vi "paste.vi"(2 "copyAry":string[][](array[string]), 3 "future event?":bool, 4 "Value":i32[](array[numeric]), 5 "ItemNames in":string[][](array[string])) -> (0 "val(sgnl)":i32[](array[numeric]), 1 "ItemNames out":string[][](array[string]))   [LabVIEW 2021]
panel:
  # "About This VI (pastes copied array to the LIST under highlighted cursor)\n- Pastes (inserts) copied array, called \"coppery\" underneath highlighted row of array \"ItemName in\" and outputs resulting array \"ItemNames out\"  \n\n*If highlighted cursor is located at the past event, it will send \"You cannot edit the current or past sequence.\" message.\n*Also, if highlighted cursor has multiple value, that is to say if multiple  lines are highlighted, it will send \"Select only one line  to add more.\" message."
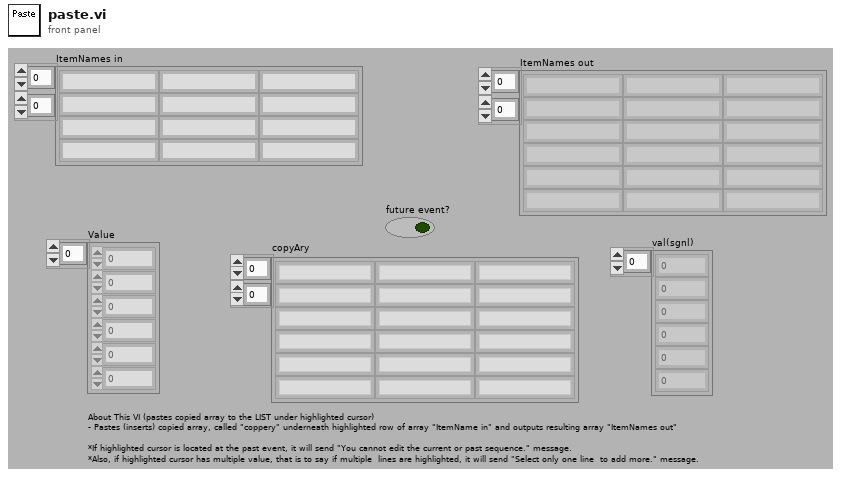
[diagram p1: front panel]
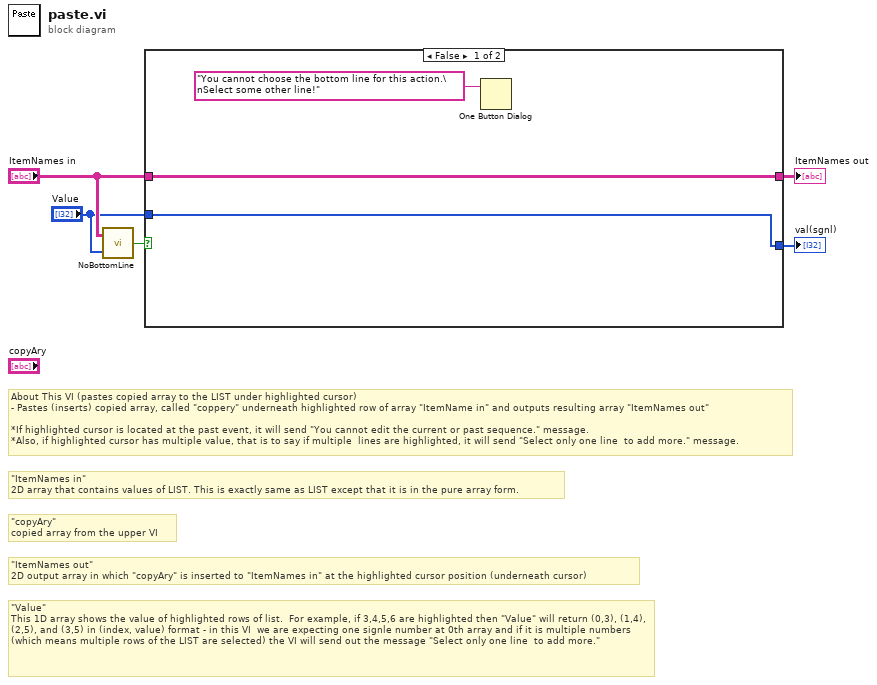
[diagram p0: block diagram]
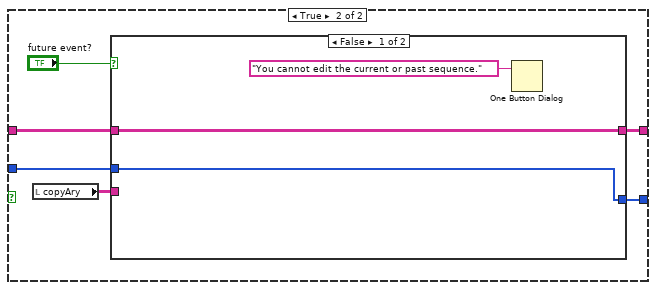
[diagram p2: hidden frame]
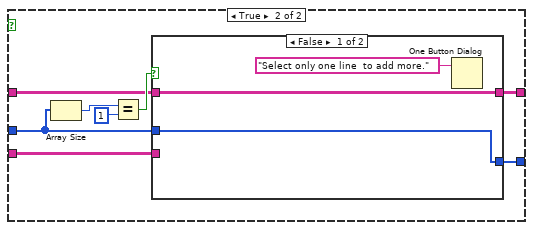
[diagram p3: hidden frame]
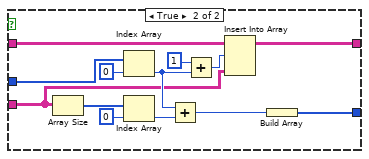
[diagram p4: hidden frame]
diagram:
  # "About This VI (pastes copied array to the LIST under highlighted cursor)\n- Pastes (inserts) copied array, called \"coppery\" underneath highlighted row of array \"ItemName in\" and outputs resulting array \"ItemNames out\"  \n\n*If highlighted cursor is located at the past event, it will send \"You cannot edit the current or past sequence.\" message.\n*Also, if highlighted cursor has multiple value, that is to say if multiple  lines are highlighted, it will send \"Select only one line  to add more.\" message."
  # "\"Value\"\nThis 1D array shows the value of highlighted rows of list.  For example, if 3,4,5,6 are highlighted then \"Value\" will return (0,3), (1,4), (2,5), and (3,5) in (index, value) format - in this VI  we are expecting one signle number at 0th array and if it is multiple numbers (which means multiple rows of the LIST are selected) the VI will send out the message \"Select only one line  to add more.\""
  # "\"ItemNames out\"\n2D output array in which \"copyAry\" is inserted to \"ItemNames in\" at the highlighted cursor position (underneath cursor)"
  # "\"copyAry\"\ncopied array from the upper VI"
  # "\"ItemNames in\"\n2D array that contains values of LIST. This is exactly same as LIST except that it is in the pure array form."
  n1 = call "NoBottomLine.vi"("Value in"="Value", "ItemNames in"="ItemNames in") -> ("no bottom?"=w4:bool)
  n2 = case shown="False" w4 {
    tunnel: "ItemNames in" -> [w8 w14]
    tunnel: "Value" -> [w6 w13]
    tunnel: [w8 w11] -> w5
    tunnel: [w6 w9] -> w1
    frame False {
      n3 = One Button Dialog(message="You cannot choose the bottom line for this action.\nSelect some other line!") -> ()  [unwired: 1 in, 1 out]
    }
    frame True {
      n4 = local read "copyAry"() -> (w10:string[][])
      n5 = case shown="False" "future event?" {
        tunnel: [w17 w22] -> w11
        tunnel: w14 -> [w17 w21]
        tunnel: w13 -> [w15 w20]
        tunnel: w10 -> [_ w19]
        tunnel: [w15 w18] -> w9
        frame False {
          n6 = One Button Dialog(message="You cannot edit the current or past sequence.") -> ()  [unwired: 1 in, 1 out]
        }
        frame True {
          n7 = Array Size(array=w20) -> (size(s)=w25:i32)
          n8 = Equal?(x=w25, y=1) -> (x = y?=w23:bool)
          n9 = case shown="False" w23 {
            tunnel: w21 -> [w27 w41]
            tunnel: [w27 w40] -> w22
            tunnel: w20 -> [w26 w33]
            tunnel: w19 -> [_ w31]
            tunnel: [w26 w30] -> w18
            frame False {
              n10 = One Button Dialog(message="Select only one line  to add more.") -> ()  [unwired: 1 in, 1 out]
            }
            frame True {
              n11 = Array Size(array=w31) -> (size(s)=w37:i32[])
              n12 = Index Array(array=w33, index=0) -> (element=w35:i32)
              n13 = Index Array(array=w37, index=0) -> (element=w34:i32)
              n14 = Add(x=w35, y=w34) -> (x+y=w32:i32)
              n15 = Add(x=1, y=w35) -> (x+y=w29:i32)
              n16 = Insert Into Array(array=w41, index (row)=w29, new element=w31) -> (w40:string[][])  [unwired: 1 in]
              n17 = Build Array(w32) -> (w30:i32[])
            }
          }
        }
      }
    }
  }
  "ItemNames out" <- w5
  "val(sgnl)" <- w1
